vi "ScratchPad_FindAllPaths.vi"(6 "path":i32[](array[numeric]), 8 "error in (no error)":errorcluster, 9 "End Vertex":i32, 10 "Start Vertex":i32, 11 "variant":variant) -> (0 "error out":errorcluster, 3 "paths":i32[][](array[numeric]))   [LabVIEW 2013, in "Graph.lvclass"]
uses:
  Graph.lvclass
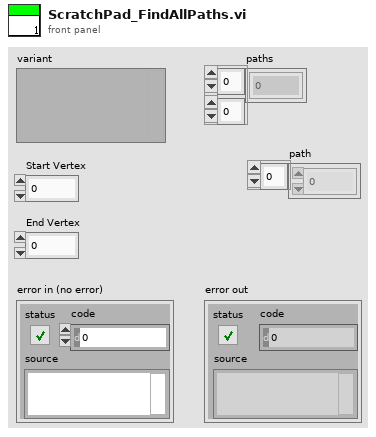
[diagram p1: front panel]
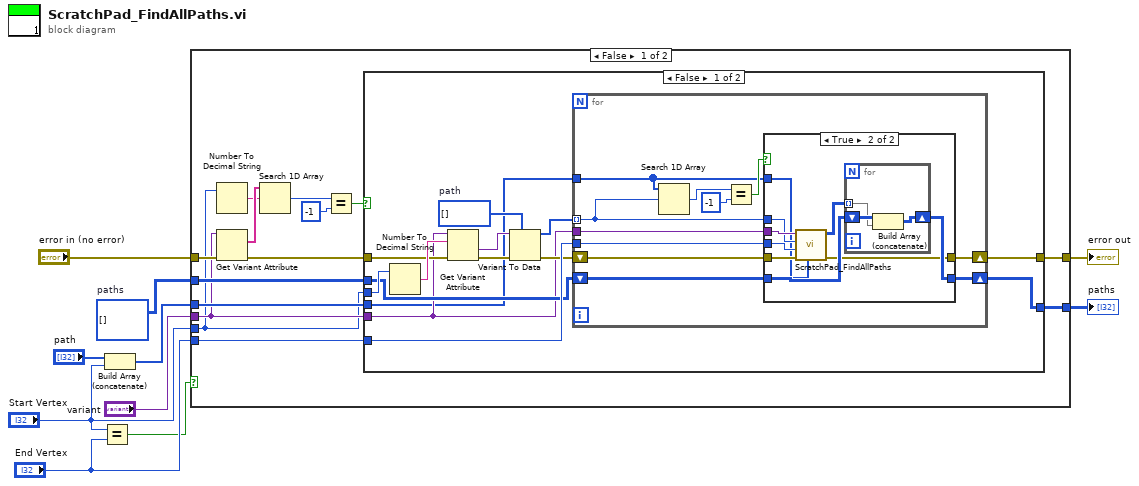
[diagram p0: block diagram]
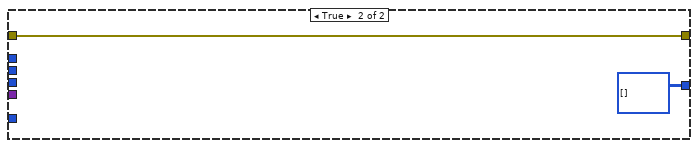
[diagram p3: hidden frame]
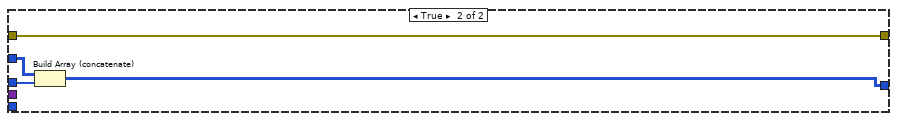
[diagram p4: hidden frame]
diagram:
  w5 = i32[][] []  # paths
  n1 = Equal?(x="Start Vertex", y="End Vertex") -> (x = y?=w6:bool)
  n2 = Build Array (concatenate)("path", "Start Vertex") -> (w1:i32[])
  n3 = case shown="False" w6 {
    tunnel: w1 -> [w24 w68]
    tunnel: [w23 w66] -> w10
    tunnel: "Start Vertex" -> [w16 _]
    tunnel: "End Vertex" -> [w22 _]
    tunnel: "error in (no error)" -> [w19 w66]
    tunnel: [w21 w67] -> w8
    tunnel: w5 -> [w20 w69]
    tunnel: "variant" -> [w17 _]
    frame False {
      n4 = Number To Decimal String(number=w16) -> (decimal integer string=w14:string)  [unwired: 1 in]
      n5 = Get Variant Attribute(Variant=w17, error in=w19) -> (names=w15:string[], error out=w18:errorcluster)  [unwired: 2 in, 2 out]
      n6 = Search 1D Array(1D array=w15, element=w14) -> (index of element=w13:i32)  [unwired: 1 in]
      n7 = Equal?(x=w13, y=-1) -> (x = y?=w11:bool)
      n8 = case shown="False" w11 {
        tunnel: w24 -> [w25 _]
        tunnel: [w38 w65] -> w23
        tunnel: w16 -> [w37 _]
        tunnel: w22 -> [w36 _]
        tunnel: w18 -> [w29 w65]
        tunnel: [w28 i32[][] [] ("paths")] -> w21
        tunnel: w20 -> [w27 _]
        tunnel: w17 -> [w26 _]
        frame False {
          w32 = i32[] []  # path
          n9 = Number To Decimal String(number=w37) -> (decimal integer string=w35:string)  [unwired: 1 in]
          n10 = Get Variant Attribute(Variant=w26, name=w35, error in=w29) -> (value=w34:variant, error out=w33:errorcluster)  [unwired: 1 in, 2 out]
          n11 = Variant To Data(error in=w33, type=w32, Variant=w34) -> (data=w31:i32[], error out=w30:errorcluster)
          n12 = for {
            tunnel: w31 -> [w44] mode=indexing
            tunnel: w25 -> [w39]
            shift-right: [w45] -> w38
            shift-left: w30 -> [w46]
            tunnel: w36 -> [w43]
            shift-right: [w41] -> w28
            shift-left: w27 -> [w42]
            tunnel: w26 -> [w40]
            n13 = Search 1D Array(1D array=w39, element=w44) -> (index of element=w48:i32)  [unwired: 1 in]
            n14 = Equal?(x=w48, y=-1) -> (x = y?=w47:bool)
            n15 = case shown="True" w47 {
              tunnel: w46 -> [w51 w56]
              tunnel: [w51 w55] -> w45
              tunnel: w44 -> [_ w54]
              tunnel: w43 -> [_ w53]
              tunnel: w42 -> [w50 w60]
              tunnel: [w50 w58] -> w41
              tunnel: w40 -> [_ w57]
              tunnel: w39 -> [_ w52]
              frame False {
              }
              frame True {
                n16 = call "ScratchPad_FindAllPaths.vi"("path"=w52, "error in (no error)"=w56, "End Vertex"=w53, "Start Vertex"=w54, "variant"=w57) -> ("error out"=w55:errorcluster, "paths"=w59:i32[][])  [unwired: 5 in]
                n17 = for {
                  shift-right: [w63] -> w58
                  shift-left: w60 -> [w62]
                  tunnel: w59 -> [w61] mode=indexing
                  n18 = Build Array (concatenate)(w62, w61) -> (w63:i32[][])
                }
              }
            }
          }
        }
        frame True {
        }
      }
    }
    frame True {
      n19 = Build Array (concatenate)(w69, w68) -> (w67:i32[][])
    }
  }
  "error out" <- w10
  "paths" <- w8
